vi "Write Standard.vi"(8 "error in (no error)":errorcluster, 10 "Standard":string, 11 "RxBN dBmHz Calculation in":refnum<class "RxBN dBmHz Calculation.lvclass">) -> (0 "error out":errorcluster, 3 "RxBN dBmHz Calculation out":refnum<class "RxBN dBmHz Calculation.lvclass">)   [LabVIEW 2018, in "SeqAuto Evaluations.lvlib" / "RxBN dBmHz Calculation.lvclass"]
uses:
  RxBN dBmHz Calculation.lvclass
  RxBN dBmHz Calculation.lvclass/RxBN dBmHz Calculation.ctl
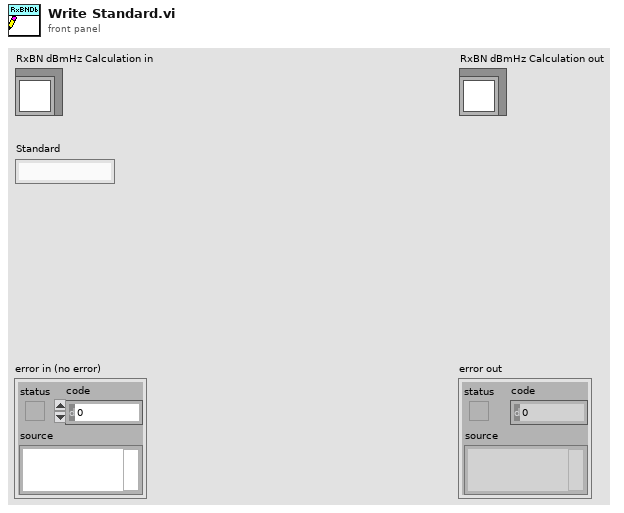
[diagram p1: front panel]
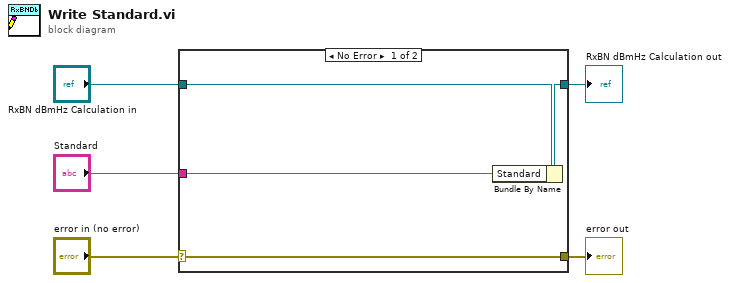
[diagram p0: block diagram]
diagram:
  n1 = case shown="No Error" "error in (no error)" {
    selector: "error in (no error)" -> [w9 w10]
    tunnel: [w9 w10] -> w4
    tunnel: [w7 w11] -> w2
    tunnel: "RxBN dBmHz Calculation in" -> [w8 w11]
    tunnel: "Standard" -> [w6 _]
    frame No Error {
      n2 = Bundle By Name(cluster=w8, "Standard"=w6) -> (w7:refnum<class "RxBN dBmHz Calculation.lvclass">)
    }
    frame Error {
    }
  }
  "error out" <- w4
  "RxBN dBmHz Calculation out" <- w2
